vi "_OLS_Main_Q02.vi"() -> ()   [LabVIEW 2024]
uses:
  Control Definitions/Def_PumpSpeed.ctl
  Control Definitions/Def TestState.ctl
  Control Definitions/DEF_PumpCtlRefs.ctl
  Control Definitions/DEF_Results.ctl
  Control Definitions/DEF_ Results3.ctl
  Control Definitions/Def_ATPStatus.ctl
  Control Definitions/DEF_TestInfo.ctl
  Control Definitions/Registry Keys.ctl
  Control Definitions/Global 2.vi
  Control Definitions/Global 1.vi
panel:
  out "vi path":path
  out "Config Path":path
  out "Laser\nOnline":bool=TRUE
  out "Report Path":path
  out "Pefump VISA Ref":refnum<visa-resource-name>
  out "Test Info":T1={"Job Number"="", "Unit Number"="", "Serial Number"="", "Technician Name"="", "Calibration Date"="Cal Date", "Calibrator"="Cal by", "Calibration Slope"="M", "Calibration Offset"="B", "Config File Name"="Cal Date"}
  out "Results":T2 {"Resistor 2" format="%.1f"; "Drain" format="%.3f"; "Resistor" format="%.1f"; "Fill" format="%.3f"}
  in  "End Prog":bool=TRUE
  out "Test Index Out":i32
  out "PumpCtlRef out":T5
  out "TEST State Out":T6
  in  "Pump Speed":T7
  out "Ch B  Sim":dbl=101.0
  out "Ch A  Sim":dbl=200.0
  out "Root Path":path=path "C:/AllenProjects/PWC-OLS"
  out "Time(ms)":dbl=1249.4499999994114
  in  "ChA":dbl(slide)=24.489795918367346 scale=0.0..1200.0
  in  "ChB":dbl(slide)=36.73469387755102 scale=0.0..1200.0
  in  "ChB +100":bool
  in  "ChA +100":bool
  in  "Check":bool
  in  "DUT":i16=1
  in  "Pump JOG":bool=TRUE
  in  "Run Test":bool
  out "Pump Online":bool=TRUE
  out "DataQ\nOnline":bool=TRUE
  in  "Level SP":dbl(slide)=8.0 scale=8.5..2.0
  in  "Level PV":dbl(slide)=7.715118932422306 scale=8.5..2.0
  out "Level":dbl=7.715118932422306 format="%.3f"
  in  "Drain":bool
  in  "Fill":bool
  in  "Simulate":bool
  out "TEST Name":string="OLR001--cal"
  out "DataQ Input":T8(graph)={"ChA Ohms"=100.83065830421491, "ChB Ohms"=100.0340857774357, "Laser (raw)"=1.9040000438690186}
  out "Time Stamp":timestamp=timestamp(3810639016.2712703 s since 1904-01-01)
  in  "stop":bool
  out "ChB Ohms":dbl=100.0340857774357 format="%.1f"
  out "ChA Ohms":dbl=100.79497115454612 format="%.1f"
  # "CHA             Resistance     Fill     Resistance   Drain"
  # "CHB           Resistance     Fill     Resistance   Drain"
  # "PUMP"
  # "Simulated Resistor In"
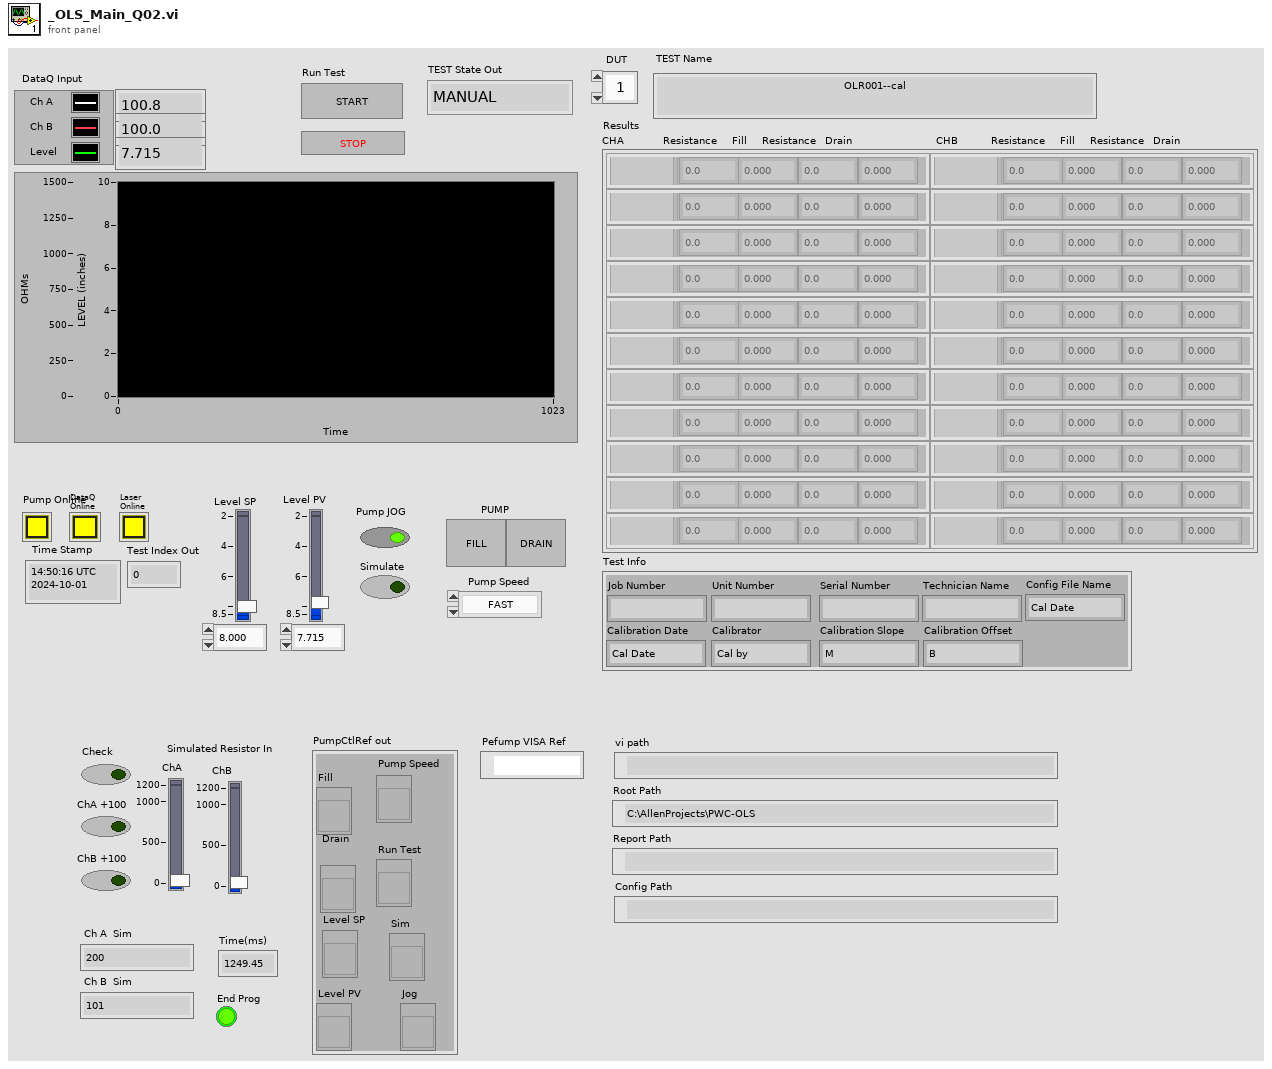
[diagram p1: front panel]
types:
  T1 = typedef "DEF_TestInfo.ctl" = cluster{"Job Number":string, "Unit Number":string, "Serial Number":string, "Technician Name":string, "Calibration Date":string, "Calibrator":string, "Calibration Slope":string, "Calibration Offset":string, "Config File Name":string}
  T2 = typedef "DEF_Results.ctl" = T3[][]
  T3 = typedef "DEF_ Results3.ctl" = cluster{"Fill":dbl, "Status":T4, "Resistor":dbl, "Drain":dbl, "Resistor 2":dbl}
  T4 = typedef "Def_ATPStatus.ctl" = i16
  T5 = typedef "DEF_PumpCtlRefs.ctl" = cluster{"Fill ":refnum<vi>, "Drain":refnum<vi>, "Level PV":refnum<vi>, "Pump Speed":refnum<vi>, "Run Test":refnum<vi>, "Sim":refnum<vi>, "Jog":refnum<vi>, "Level SP":refnum<vi>}
  T6 = typedef "Def TestState.ctl" = enum16{"MANUAL", "Start", "Pre-Fill", "Pre-Fill Measure", "Pre-Drain", "Pre-Drain Measure", "Init-Record", "Load Fill Spec", "Filling Hi", "Wait1", "Record Fill", "Load Drain Spec", "Draining Lo", "Wait2", "Record Drain", "Empty", "Done"}
  T7 = typedef "Def_PumpSpeed.ctl" = enum16{"FAST", "SLOW", "CREEP", "STOP"}
  T8 = cluster{"ChA Ohms":dbl, "ChB Ohms":dbl, "Laser (raw)":dbl}
  T9 = typedef "Registry Keys.ctl" = enum16{"Report Files Key", "Config Files Key"}
  T10 = cluster{"Pump Online":refnum<vi>, "DataQ\nOnline":refnum<vi>, "Laser\nOnline":refnum<vi>, "ChA Ohms":refnum<vi>, "ChB Ohms":refnum<vi>}
  T11 = typedef "DEF_FullConfig.ctl" = cluster{"Bench Params":T12, "Test Params":dbl[][], "Pump Params":T13, "DataQ Params":T14, "Pump Control Ref":T5, "Bench Status":T15}
  T12 = typedef "DEF_BenchParams.ctl" = cluster{"Relative Root Name":string, "Values":cluster{"Step Levels":dbl, "Resistor Tolerence":dbl, "Sample Rate":dbl, "Resistor":dbl, "Wait Time":dbl}, "Report Template path":path, "Test Type":string, "Config File Name":string, "Config 2 Use":string, "Skip Pre Lube":bool}
  T13 = typedef "DEF_PumpParams.ctl" = cluster{"Empty Inches":dbl, "Full Inches":dbl, "RNG_SLOW":dbl, "RNG_CREEP":dbl, "RNG_STOP ":dbl, "VISA resource name":refnum<visa-resource-name>, "SPD_SLOW":i32, "SPD_CREEP":i32, "SPD_FAST":i32, "Zero template":path, "zero  Settle sec":i32, "Laser Slope":sgl, "Laser Offset":sgl, "Sim Fill Rate":sgl, "Cal Date":string, "Cal Technician":string}
  T14 = typedef "DEF_DataqParams.ctl" = cluster{"Visa Name":string, "Num Chan":i32, "Cal Coef":cluster{"M":dbl, "B":dbl}[], "Scale ":i32, "Cal Date":string, "Cal Technicain":string}
  T15 = typedef "DEF_BenchStatus.ctl" = cluster{"Pump Status":refnum<vi>, "Dataq Status":refnum<vi>, "LaserStatus":refnum<vi>, "ChA Ohms":refnum<vi>, "ChB Ohms":refnum<vi>}
  T16 = enum16{"MANUAL", "Start", "Filling", "FULL", "Draining", "EMPTY", "Done"}
  T17 = typedef "DEF_LevelOut.ctl" = cluster{"Laser ":cluster{"Raw":sgl, "Scaled":dbl}, "Level PV":dbl, "Fill":bool, "Drain":bool}
  T18 = typedef "DEF_SpecsOut.ctl" = cluster{"aSpecsTable":T19[], "Pump CtlRef In":T5, "TEST State Out":T6, "TEST Index":i32, "Drain!Fill":bool}
  T19 = typedef "Def Spec RNG.ctl" = cluster{"Specs":dbl[], "LUT Status":T20}
  T20 = typedef "Ded LUT_Status.ctl" = cluster{"ChA/!ChB":bool, "Drain/!Fill":bool, "In Range?":bool, "Switch Range?":bool, "Measure R?":bool, "Vaild R?":bool, "Index(n)":i32, "Index(n)-1":i32, "Index Max":i32, "Index(n-1)":i32}
  T21 = typedef "Def Measure.ctl" = cluster{"ChA R":dbl, "ChB R":dbl, "Level PV":dbl}
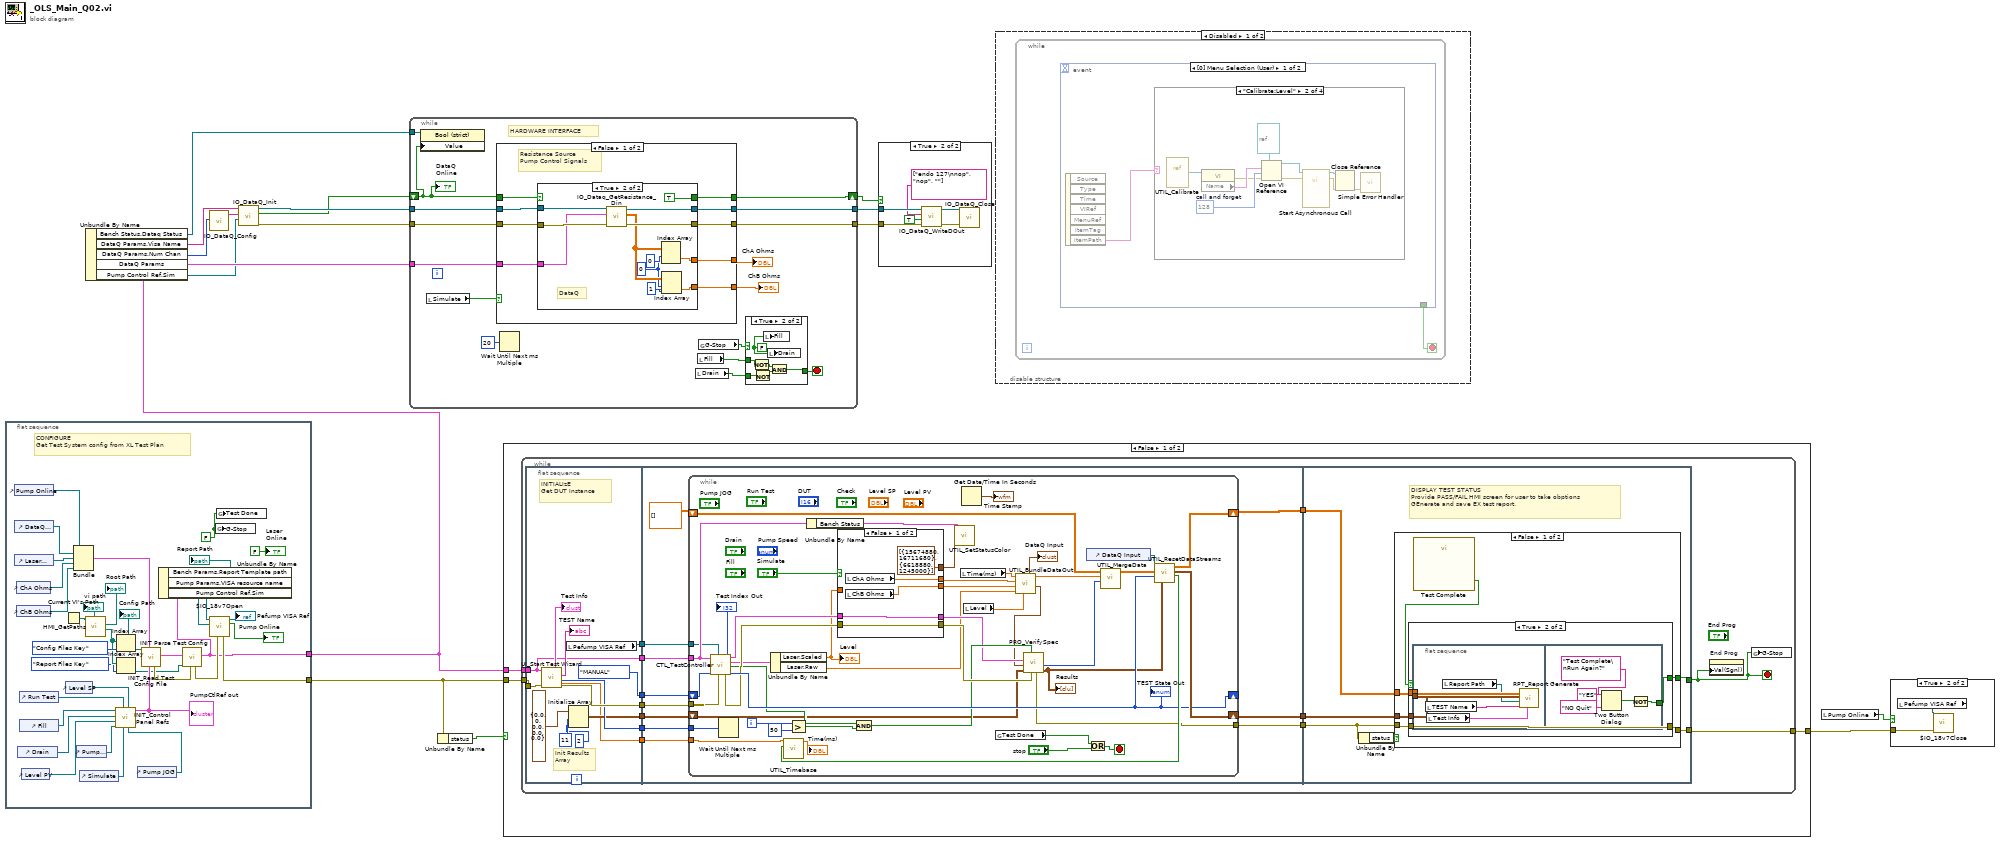
[diagram p0: block diagram]
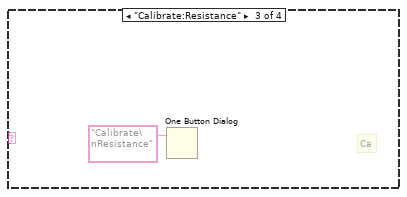
[diagram p5: hidden frame]
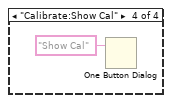
[diagram p6: hidden frame]
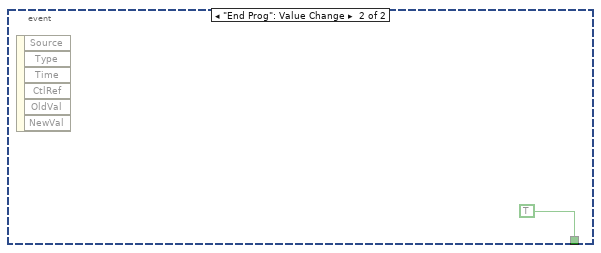
[diagram p7: hidden frame]
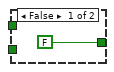
[diagram p9: hidden frame]
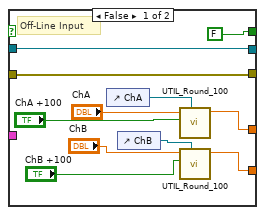
[diagram p10: hidden frame]
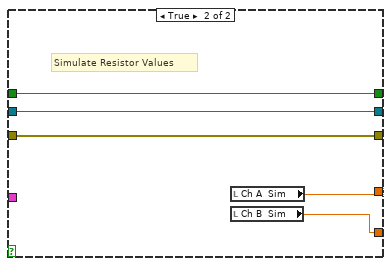
[diagram p11: hidden frame]
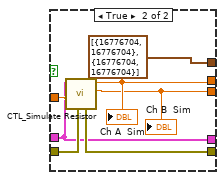
[diagram p12: hidden frame]
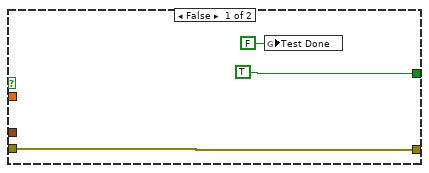
[diagram p13: hidden frame]
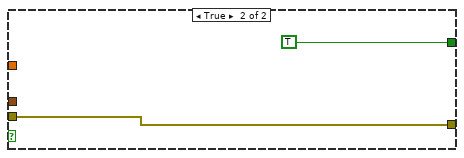
[diagram p14: hidden frame]
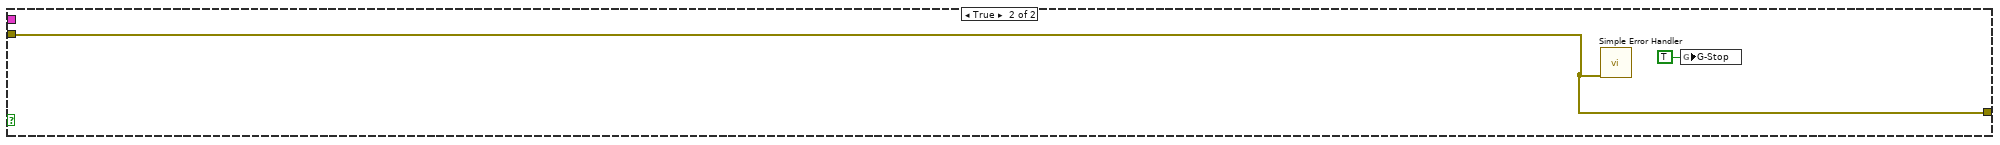
[diagram p15: hidden frame]
diagram:
  n1 = flat-sequence {
    tunnel: [w27] -> w16
    tunnel: [w23] -> w15
    frame #0 {
      w43 = FALSE ("G-Stop")
      # "CONFIGURE\nGet Test System config from XL Test Plan"
      n2 = control-ref of="Pump Online"() -> (w51:refnum<vi>)
      n3 = control-ref of="Laser\nOnline"() -> (w29:refnum<vi>)
      n4 = control-ref of="DataQ\nOnline"() -> (w45:refnum<vi>)
      n5 = control-ref of="ChA Ohms"() -> (w19:refnum<vi>)
      n6 = control-ref of="ChB Ohms"() -> (w18:refnum<vi>)
      n7 = control-ref of="Drain"() -> (w52:refnum<vi>)
      n8 = control-ref of="Run Test"() -> (w48:refnum<vi>)
      n9 = control-ref of="Fill"() -> (w49:refnum<vi>)
      n10 = control-ref of="Level PV"() -> (w50:refnum<vi>)
      n11 = Current VI's Path() -> (path=w24:path)
      n12 = control-ref of="Level SP"() -> (w44:refnum<vi>)
      n13 = Bundle("Pump Online"=w51, "DataQ\nOnline"=w45, "Laser\nOnline"=w29, "ChA Ohms"=w19, "ChB Ohms"=w18) -> (w38:T10)  [unwired: 1 in]
      n14 = control-ref of="Pump Speed"() -> (w41:refnum<vi>)
      n15 = control-ref of="Simulate"() -> (w47:refnum<vi>)
      n16 = call "HMI_GetPaths.vi"("Main Root Path"=w24) -> ("Default Paths"=w22:path[], "Root Path"=→"Root Path":path, "vi path"=→"vi path":path)  [unwired: 8 in]
      n17 = Index Array(array=w22, index=Registry_Keys."Config Files Key" ("Reg Key")) -> (element=w39:path)
      "Config Path" <- w39
      n18 = Index Array(array=w22, index=Registry_Keys."Report Files Key" ("Reg Key")) -> (element=w20:path)
      n19 = control-ref of="Pump JOG"() -> (w46:refnum<vi>)
      n20 = call "INIT_Control Panel Refs.vi"("Jog"=w46, "Level SP"=w44, "Sim"=w47, "Run Test"=w48, "Pump Speed"=w41, "Level PV"=w50, "Drain"=w52, "Fill"=w49) -> ("PumpCtlRef out"=w37:T5)  [unwired: 3 in]
      "PumpCtlRef out" <- w37
      n21 = call "INIT_Read Test Config File.vi"("Pump Control Ref"=w37, "Bench Status"=w38, "Path"=w39) -> ("FullConfig"=w35:T11, "error out"=w36:errorcluster)  [unwired: 7 in]
      n22 = call "INIT Parse Test Config.vi"("error in"=w36, "Report Path"=w20, "Full Config In"=w35) -> ("Full Config Out"=w23:T11, "error out"=w28:errorcluster)  [unwired: 7 in]
      n23 = Unbundle By Name(w23) -> ("Bench Params.Report Template path"=→"Report Path":path, "Pump Params.VISA resource name"=w34:refnum<visa-resource-name>, "Pump Control Ref.Sim"=w31:refnum<vi>)
      n24 = call "$IO_18v7Open.vi"("error in"=w28, "Pump Control Ref.Sim"=w31, "Runtime VISA name"=w34) -> ("Connected"=→"Pump Online":bool, "VISA Refnum out"=→"Pefump VISA Ref":refnum<visa-resource-name>, "error out"=w27:errorcluster)  [unwired: 6 in]
      n25 = global write "Global 1.vi" "G-Stop"(w43) -> ()
      n26 = global write "Global 2.vi" "Test Done"(w43) -> ()
      "Laser\nOnline" <- FALSE ("Laser\nStatus")
    }
  }
  n27 = Unbundle By Name(w15) -> ("Bench Status.Dataq Status"=w1:refnum<vi>, "DataQ Params.Visa Name"=w7:string, "DataQ Params.Num Chan"=w8:i32, "DataQ Params"=w6:T14, "Pump Control Ref.Sim"=w4:refnum<vi>)
  n28 = call "IO_DataQ_Config.vi"("Num Chan"=w8) -> ("Init Message"=w14:string[])  [unwired: 10 in]
  n29 = call "IO_DataQ_Init.vi"("Pump Control Ref.Sim"=w4, "Command\nList"=w14, "RunTime VISA name"=w7) -> ("error out"=w12:errorcluster, "Connected?"=w11:bool, "VISA resource name out"=w13:refnum<visa-resource-name>)  [unwired: 6 in]
  n30 = while {
    tunnel: w13 -> [w66]
    tunnel: w12 -> [w65]
    tunnel: [w63] -> w10
    tunnel: [w64] -> w9
    shift-right: [w62] -> w3
    shift-left: w11 -> [w53]
    tunnel: w6 -> [w55]
    tunnel: w1 -> [w54]
    stop <- w59 stop-if-true
    # "HARDWARE INTERFACE"
    n31 = property class="Bool (strict)"(reference=w54, "Value"=w53) -> ()  [unwired: 1 in, 2 out]
    n32 = local read "Simulate"() -> (w61:bool)
    n33 = case shown="False" w61 {
      tunnel: [w84 w109] -> w67
      tunnel: [w83 w108] -> w56
      tunnel: w66 -> [w77 w111]
      tunnel: w65 -> [w78 w110]
      tunnel: [w82 w110] -> w64
      tunnel: [w81 w111] -> w63
      tunnel: [w80 w112] -> w62
      tunnel: w53 -> [w79 w112]
      tunnel: w55 -> [w76 _]
      frame False {
        # "Resistance Source\nPump Control Signals"
        n34 = case shown="True" w79 {
          tunnel: [w88 w104] -> w84
          tunnel: [w89 w101] -> w83
          tunnel: [w90 w107] -> w81
          tunnel: [w91 w106] -> w82
          tunnel: [FALSE TRUE] -> w80
          tunnel: w78 -> [w91 w97]
          tunnel: w77 -> [w90 w98]
          tunnel: w76 -> [_ w96]
          frame False {
            # "Off-Line Input"
            n35 = control-ref of="ChA"() -> (w87:refnum<vi>)
            n36 = control-ref of="ChB"() -> (w85:refnum<vi>)
            n37 = call "UTIL_Round_100.vi"("Num Refnum"=w87, "100"="ChA +100", "IN"="ChA") -> ("OUT"=w89:dbl)  [unwired: 8 in]
            n38 = call "UTIL_Round_100.vi"("Num Refnum"=w85, "100"="ChB +100", "IN"="ChB") -> ("OUT"=w88:dbl)  [unwired: 8 in]
          }
          frame True {
            w100 = 0 ("disabled index (col)")
            # "DataQ"
            n39 = call "IO_Dataq_GetResistance_Din.vi"("error in (no error)"=w97, "Dataq Params"=w96, "VISA Refnum in"=w98) -> ("error out"=w106:errorcluster, "Analog"=w102:dbl[][], "VISA Refnum out"=w107:refnum<visa-resource-name>)  [unwired: 5 in, 1 out]
            n40 = Index Array(array=w102, index (row)=0 ("index"), index (col)=w100) -> (element=w101:dbl)
            n41 = Index Array(array=w102, index (row)=w100, index (col)=1 ("index")) -> (element=w104:dbl)
          }
        }
      }
      frame True {
        # "Simulate Resistor Values"
        n42 = local read "Ch A  Sim"() -> (w108:dbl)
        n43 = local read "Ch B  Sim"() -> (w109:dbl)
      }
    }
    "ChA Ohms" <- w56
    "ChB Ohms" <- w67
    n44 = Wait Until Next ms Multiple(millisecond multiple=u32 20) -> ()  [unwired: 1 out]
    n45 = local read "Drain"() -> (w57:bool)
    n46 = local read "Fill"() -> (w58:bool)
    n47 = global read "Global 1.vi" "G-Stop"() -> (w60:bool)
    n48 = case shown="True" w60 {
      tunnel: [FALSE w71] -> w59
      tunnel: w58 -> [_ w73]
      tunnel: w57 -> [_ w70]
      frame False {
      }
      frame True {
        w75 = FALSE
        n49 = Not(x=w73) -> (.not. x?=w74:bool)
        n50 = Not(x=w70) -> (.not. x?=w72:bool)
        n51 = local write "Fill"(w75) -> ()
        n52 = local write "Drain"(w75) -> ()
        n53 = And(x=w74, y=w72) -> (x .and. y?=w71:bool)
      }
    }
    "DataQ\nOnline" <- w53
  }
  n54 = Unbundle By Name(w16) -> ("status"=w17:bool)
  n55 = case shown="False" w17 {
    tunnel: w16 -> [w115 w242]
    tunnel: [w114 w242] -> w5
    tunnel: w15 -> [w113 _]
    frame False {
      n56 = while {
        tunnel: w115 -> [w126]
        tunnel: [w120] -> w114
        tunnel: w113 -> [w118]
        stop <- w116 stop-if-true
        n57 = flat-sequence {
          tunnel: [w140] -> w128
          tunnel: [w141] -> w127
          tunnel: w126 -> [w142]
          tunnel: [w131] -> w125
          tunnel: [T16."MANUAL" ("TEST STATUS Out")] -> w124
          tunnel: [w136] -> w123
          tunnel: [w135] -> w119
          tunnel: w118 -> [w131]
          tunnel: [w130] -> w117
          tunnel: [w147] -> w129
          tunnel: w128 -> [w152]
          tunnel: w127 -> [w153]
          tunnel: w125 -> [w144]
          tunnel: w124 -> [w145]
          tunnel: w123 -> [w151]
          tunnel: [w150] -> w122
          tunnel: [w149] -> w121
          tunnel: w119 -> [w148]
          tunnel: w117 -> [w143]
          tunnel: w129 -> [w216]
          tunnel: [w215] -> w116
          tunnel: [w213] -> w120
          tunnel: w122 -> [w212]
          tunnel: w121 -> [w211]
          frame #0 {
            # "Init Results\nArray"
            # "INITIALIzE\nGet DUT Instance"
            n58 = call "UI_Start Test Wizard.vi"("error in (no error)"=w142, "Full Config"=w131) -> ("error out"=w141:errorcluster, "Time Base mS"=w140:i32, "Title"=→"TEST Name":string, "Sample Rate"=w135:dbl, "Test Info"=→"Test Info":T1)  [unwired: 3 in]
            n59 = local read "Pefump VISA Ref"() -> (w130:refnum<visa-resource-name>)
            n60 = Initialize Array(T3 {"Fill"=0.0, "Status"=0, "Resistor"=0.0, "Drain"=0.0, "Resistor 2"=0.0} ("Cluster 2"), 11 ("dimension size"), 2 ("dimension size")) -> (w136:T3[][])
          }
          frame #1 {
            n61 = while {
              tunnel: w152 -> [w197]
              tunnel: w153 -> [w188]
              tunnel: [w175] -> w147
              shift-right: [w182] -> w149
              shift-left: w151 -> [w161]
              tunnel: w148 -> [w187]
              shift-right: [w183] -> w150
              shift-left: dbl[][] [] ("Array") -> [w170]
              shift-right: [w179] -> _
              shift-left: w145 -> [w178]
              tunnel: w144 -> [w159]
              tunnel: w143 -> [w155]
              i -> [w186]
              stop <- w194 stop-if-true
              n62 = call "CTL_TestController.vi"("error in (no error)"=w188, "VISA Refnum In"=w155, "TEST State In"=w178, "FullConfig"=w159) -> ("TEST State Out"=w179:T6, "Enable"=w163:bool, "Level Out"=w158:T17, "Specs Out"=w165:T18, "error out"=w164:errorcluster, "Test Index Out"=→"Test Index Out":i32)  [unwired: 2 in]
              "TEST State Out" <- w179
              n63 = Wait Until Next ms Multiple(millisecond multiple=w197) -> ()  [unwired: 1 out]
              n64 = Unbundle By Name(w158) -> ("Laser.Scaled"=w156:dbl, "Laser.Raw"=w157:sgl)
              "Level" <- w156
              n65 = Greater?(x=w186, y=50) -> (0:w184:bool)
              n66 = Unbundle By Name(w159) -> ("Bench Status"=w195:T15)
              n67 = case shown="False" "Simulate" {
                tunnel: w164 -> [w203 w206]
                tunnel: [w203 w209] -> w177
                tunnel: [cluster{u32, u32}[] [{15674880, 16711680}, {6618880, 1245000}] ("Normal") cluster{u32, u32}[] [{16776704, 16776704}, {16776704, 16776704}] ("Sim Color")] -> w196
                tunnel: [w201 w208] -> w190
                tunnel: [w200 w207] -> w189
                tunnel: w165 -> [w199 w204]
                tunnel: w156 -> [_ w205]
                tunnel: [w199 w204] -> w174
                frame False {
                  n68 = local read "ChA Ohms"() -> (w201:dbl)
                  n69 = local read "ChB Ohms"() -> (w200:dbl)
                }
                frame True {
                  n70 = call "CTL_Simulate Resistor.vi"("error in (no error)"=w206, "Level IN"=w205, "Specs IN"=w204) -> ("Ch B  Ohms"=w207:dbl, "Ch A  Ohms"=w208:dbl, "error out"=w209:errorcluster)  [unwired: 6 in]
                  "Ch A  Sim" <- w208
                  "Ch B  Sim" <- w207
                }
              }
              n71 = And(x=w163, y=w184) -> (x .and. y?=w176:bool)
              n72 = call "UTIL_SetStatusColor.vi"("Colors [4] in"=w196, "Bench Status"=w195) -> ()  [unwired: 10 in]
              n73 = local read "Time(ms)"() -> (w191:dbl)
              n74 = Get Date/Time In Seconds() -> (seconds since 1Jan1904=→"Time Stamp":timestamp)
              n75 = local read "Level"() -> (w166:dbl)
              n76 = global read "Global 2.vi" "Test Done"() -> (w192:bool)
              n77 = call "UTIL_BundleDataOut.vi"("Level PV"=w166, "Laser (raw)"=w157, "ChB Ohms"=w189, "ChA Ohms"=w190, "Time (ms)"=w191) -> ("Measure"=w173:T21, "Data Out"=w172:dbl[], "Chart Data"=→"DataQ Input":T8)  [unwired: 3 in, 1 out]
              n78 = call "PRO_VerifySpec.vi"("error in (no error)"=w177, "Enable"=w176, "Results in"=w161, "Measure In"=w173, "Specs In"=w174) -> ("Results out"=w160:T2, "Status Code"=w171:i32, "error out"=w175:errorcluster)  [unwired: 4 in]
              "Results" <- w160
              n79 = control-ref of="DataQ Input"() -> (w167:refnum<vi>)
              n80 = Or(x=w192, y="stop") -> (x .or. y?=w194:bool)
              n81 = call "UTIL_MergeData.vi"("Status Code"=w171, "New Data"=w172, "Data In"=w170) -> ("Data out"=w169:dbl[][])  [unwired: 8 in]
              n82 = call "UTIL_ResetDataStreams.vi"("Results in"=w160, "TEST State Out"=w179, "Data in"=w169, "WaveformChart in"=w167) -> ("Value (Signaling)"=w180:bool, "Results out"=w182:T2, "Array"=w183:dbl[][])  [unwired: 5 in]
              n83 = call "UTIL_Timebase.vi"("Reset"=w180, "Sample Rate"=w187) -> ("Time(ms)"=→"Time(ms)":dbl)  [unwired: 9 in]
            }
          }
          frame #2 {
            # "DISPLAY TEST STATUS\nProvide PASS/FAIL HMI screen for user to take obptions\nGEnerate and save EX test report."
            n84 = Unbundle By Name(w216) -> ("status"=w214:bool)
            n85 = case shown="False" w214 {
              tunnel: w216 -> [w220 w240]
              tunnel: [w221 TRUE] -> w215
              tunnel: [w219 w240] -> w213
              tunnel: w212 -> [w218 _]
              tunnel: w211 -> [w217 _]
              frame False {
                n86 = call "Test Complete"() -> ("SAVE"=w222:bool)  [unwired: 18 in, 1 out]
                n87 = case shown="True" w222 {
                  tunnel: [TRUE w226] -> w221
                  tunnel: w220 -> [w224 w229]
                  tunnel: [w224 w229] -> w219
                  tunnel: w218 -> [_ w228]
                  tunnel: w217 -> [_ w227]
                  frame False {
                    n88 = global write "Global 2.vi" "Test Done"(FALSE ("Test Done")) -> ()
                  }
                  frame True {
                    n89 = flat-sequence {
                      tunnel: w228 -> [w234]
                      tunnel: w227 -> [w231]
                      tunnel: [w235] -> w226
                      frame #0 {
                        n90 = local read "TEST Name"() -> (w233:string)
                        n91 = local read "Test Info"() -> (w232:T1)
                        n92 = local read "Report Path"() -> (w230:path)
                        n93 = call "RPT_Report Generate.vi"("Test Info"=w232, "Report Name"=w233, "template"=w230, "Results IN"=w231, "Wave Data"=w234) -> ()  [unwired: 7 in]
                      }
                      frame #1 {
                        n94 = Two Button Dialog(message="Test Complete\nRun Again?", 1:"NO Quit" ("F button name (\"Cancel\")"), 2:"YES" ("T button name (\"OK\")")) -> (T button?=w236:bool)
                        n95 = Not(x=w236) -> (.not. x?=w235:bool)
                      }
                    }
                  }
                }
              }
              frame True {
              }
            }
          }
        }
        n96 = property on="End Prog" class="Bool (strict)"("Val(Sgnl)"=w116) -> ()  [unwired: 2 in, 2 out]
        n97 = global write "Global 1.vi" "G-Stop"(w116) -> ()
      }
    }
    frame True {
      n98 = call <vilib>:"Simple Error Handler.vi"("error in (no error)"=w242) -> ()  [unwired: 4 in, 5 out]
      n99 = global write "Global 1.vi" "G-Stop"(TRUE ("G-Stop")) -> ()
    }
  }
  n100 = case shown="True" w3 {
    tunnel: w10 -> [_ w249]
    tunnel: w9 -> [_ w247]
    frame False {
    }
    frame True {
      n101 = call "IO_DataQ_WriteDOut.vi"("error in (no error)"=w247, "Msg Active"=TRUE, "Message"=string[] ["endo 127\nnop", "nop", ""], "VISA Refnum in"=w249) -> ("error out"=w246:errorcluster, "VISA Refnum out"=w248:refnum<visa-resource-name>)  [unwired: 6 in]
      n102 = call "IO_DataQ_Close.vi"("error in"=w246, "VISA resource name"=w248) -> ()  [unwired: 10 in]
    }
  }
  n103 = disable-structure shown="Disabled" {
    frame Disabled {
      n104 = while {
        stop <- w250 stop-if-true
        n105 = event shown="[0] Menu Selection (User)" {
          selector: _ -> [_ _]
          dyn-events: _ -> [_ _]
          timeout: _ -> [_ _]
          tunnel: [_ TRUE] -> w250
          event Menu Selection (User) {
            n106 = event-data() -> ("ItemPath"=w251:string)  [unwired: 1 in, 6 out]
            n107 = case shown="\"Calibrate:Level\"" w251 {
              frame "False", Default {
              }
              frame "Calibrate:Level" {
                w262 = 128  # call and forget
                n108 = vi-ref "UTIL_Calibrate.vi"() -> (w255:refnum<vi>)
                n109 = property class="VI"(reference=w255) -> (error out=w253:errorcluster, "Name"=w254:string)  [unwired: 1 in, 1 out]
                n110 = Open VI Reference(type specifier VI Refnum (for type only)=refnum<vi> refnum, vi path=w254, options=w262, error in (no error)=w253) -> (vi reference=w260:refnum<vi>, error out=w259:errorcluster)  [unwired: 2 in]
                n111 = call-by-ref "Start Asynchronous Call"(reference=w260, error in=w259) -> (reference out=w257:refnum<vi>, error out=w258:errorcluster, "Digital in"=w252:refnum<vi>)  [unwired: 10 in, 1 out]
                n112 = Close Reference(reference=w257, error in (no error)=w258) -> (error out=w256:errorcluster)
                n113 = call <vilib>:"Simple Error Handler.vi"("error in (no error)"=w256) -> ()  [unwired: 4 in, 5 out]
              }
              frame "Calibrate:Resistance" {
                # "Ca"
                n114 = One Button Dialog(message="Calibrate\nResistance") -> ()  [unwired: 1 in, 1 out]
              }
              frame "Calibrate:Show Cal" {
                n115 = One Button Dialog(message="Show Cal") -> ()  [unwired: 1 in, 1 out]
              }
            }
          }
          event "End Prog": Value Change {
            n116 = event-data() -> ()  [unwired: 1 in, 6 out]
          }
        }
      }
    }
    frame Enabled {
    }
  }
  n117 = local read "Pump Online"() -> (w2:bool)
  n118 = case shown="True" w2 {
    tunnel: w5 -> [_ w267]
    frame False {
    }
    frame True {
      n119 = local read "Pefump VISA Ref"() -> (w266:refnum<visa-resource-name>)
      n120 = call "$IO_18v7Close.vi"("error in (no error)"=w267, "VISA Refnum in"=w266) -> ()  [unwired: 10 in]
    }
  }
